vi "test.vi"() -> ()   [LabVIEW 2019]
uses:
  Settings.ctl
  <vilib>/DAQmx/write.llb/DAQmx Write (Analog DBL 1Chan 1Samp).vi
  <vilib>/DAQmx/create/channels.llb/DAQmx Create Channel (AO-Voltage-Basic).vi
  <vilib>/DAQmx/configure/timing.llb/DAQmx Timing (Sample Clock).vi
  <vilib>/DAQmx/miscellaneous.llb/DAQmx Fill In Error Info.vi
  <resource>/objmgr/daqmx.rc
panel:
  in  "rate":dbl=1000.0 format="%0.2f"
  in  "stop":bool
  in  "Sampling Rate":T1 format="%#_9f"
  in  "# Samples in":T1 format="%#_9f"
  in  "Strength (V)":dbl=5.0
  in  "Delay End (ms)":i32=52
  in  "Delay (ms)":dbl=20.0
  in  "Width of pulse (ms)":dbl=70.0
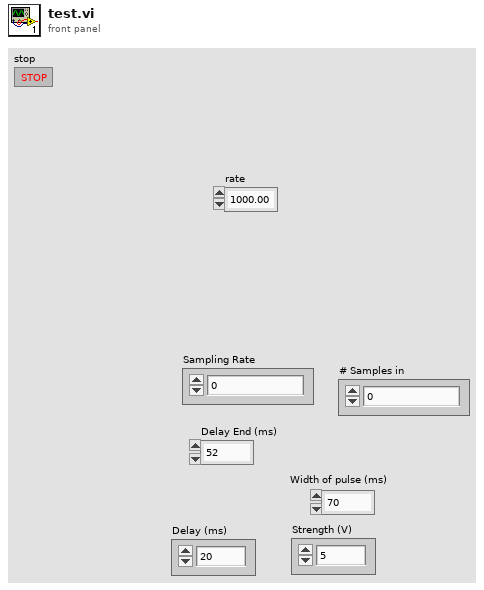
[diagram p1: front panel]
types:
  T1 = typedef "Settings.ctl" = dbl
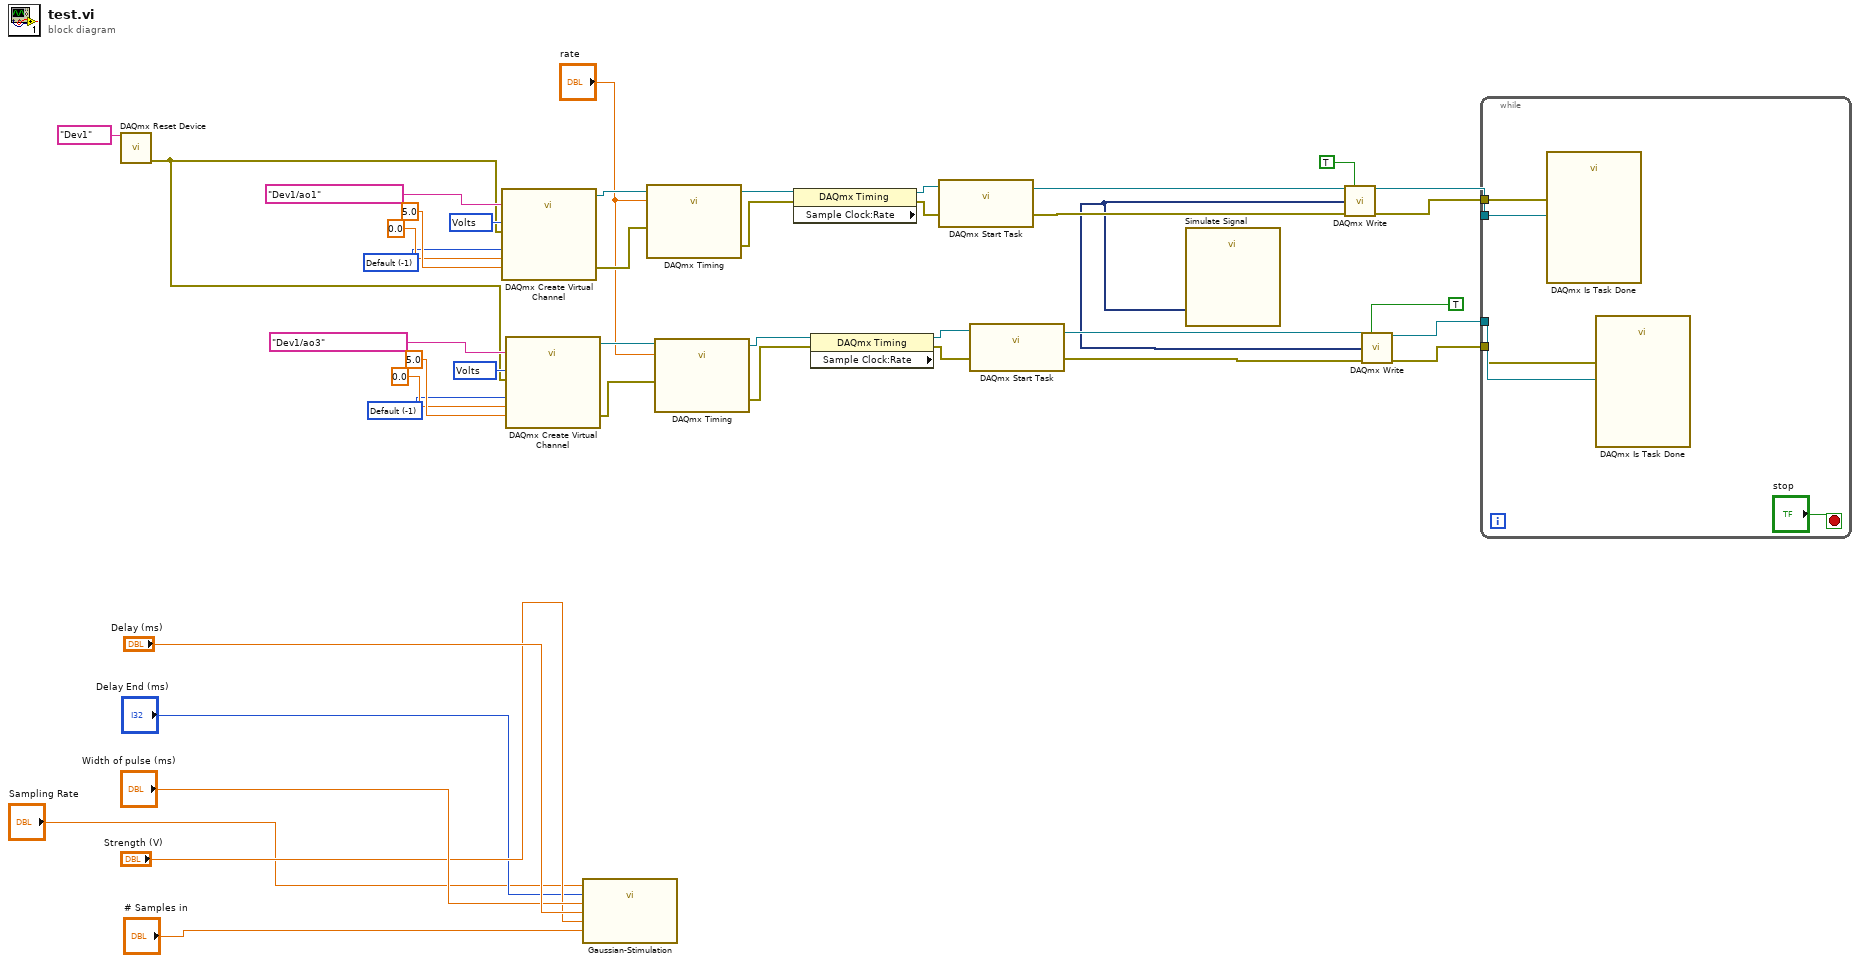
[diagram p0: block diagram]
diagram:
  w23 = 10348 items=["Volts"=10348, "From Custom Scale"=10065] ("units")
  w26 = -1 items=["Default"=-1, "RSE"=10083, "Differential"=10106, "Pseudodifferential"=12529] ("output terminal configuration")
  w36 = 10348 items=["Volts"=10348, "From Custom Scale"=10065] ("units")
  w39 = -1 items=["Default"=-1, "RSE"=10083, "Differential"=10106, "Pseudodifferential"=12529] ("output terminal configuration")
  n1 = call <vilib>:"DAQmx Reset Device.vi"("device in"=tag "Dev1") -> ("error out"=w22:errorcluster)  [unwired: 14 in]
  n2 = call-poly <vilib>:"DAQmx Create Virtual Channel.vi"("maximum value"=5.0, "minimum value"=0.0, "output terminal configuration"=w26, "physical channels"=tag "Dev1/ao1", "units"=w23, "error in"=w22) -> ("task out"=w15:refnum<k21>, "error out"=w14:errorcluster)  [unwired: 8 in]
  n3 = call-poly <vilib>:"DAQmx Create Virtual Channel.vi"("maximum value"=5.0, "minimum value"=0.0, "output terminal configuration"=w39, "physical channels"=tag "Dev1/ao3", "units"=w36, "error in"=w22) -> ("task out"=w9:refnum<k21>, "error out"=w8:errorcluster)  [unwired: 8 in]
  n4 = call "Gaussian-Stimulation.vi"("Strength (V)"="Strength (V)", "Delay (ms)"="Delay (ms)", "# Samples in"="# Samples in", "Width of pulse (ms)"="Width of pulse (ms)", "Delay End (ms)"="Delay End (ms)", "Sampling Rate"="Sampling Rate") -> ()  [unwired: 1 in, 5 out]
  n5 = call-poly <vilib>:"DAQmx Timing.vi"("task/channels in"=w15, "rate"="rate", "error in"=w14) -> ("task out"=w13:refnum<k21>, "error out"=w12:errorcluster)  [unwired: 4 in, 7 out]
  n6 = call-poly <vilib>:"DAQmx Timing.vi"("task/channels in"=w9, "rate"="rate", "error in"=w8) -> ("task out"=w7:refnum<k21>, "error out"=w6:errorcluster)  [unwired: 4 in, 7 out]
  n7 = property class="DAQmx Timing" props=["Sample Clock:Rate"](reference=w13, error in=w12) -> (reference out=w11:refnum<k21>, error out=w10:errorcluster)  [unwired: 1 out]
  n8 = property class="DAQmx Timing" props=["Sample Clock:Rate"](reference=w7, error in=w6) -> (reference out=w5:refnum<k21>, error out=w4:errorcluster)  [unwired: 1 out]
  n9 = call <vilib>:"DAQmx Start Task.vi"("task/channels in"=w11, "error in"=w10) -> ("task out"=w25:refnum<k21>, "error out"=w24:errorcluster)  [unwired: 12 in]
  n10 = call <vilib>:"DAQmx Start Task.vi"("task/channels in"=w5, "error in"=w4) -> ("task out"=w38:refnum<k21>, "error out"=w37:errorcluster)  [unwired: 12 in]
  n11 = call "Simulate Signal"() -> ("Sine"=w20:dynamicdata)  [unwired: 6 in, 9 out]
  n12 = call-poly <vilib>:"DAQmx Write.vi"("task/channels in"=w25, "auto start"=TRUE, "data"=w20, "error in"=w24) -> ("task out"=w17:refnum<k21>, "error out"=w16:errorcluster)  [unwired: 9 in, 1 out]
  n13 = call-poly <vilib>:"DAQmx Write.vi"("task/channels in"=w38, "auto start"=TRUE, "data"=w20, "error in"=w37) -> ("task out"=w3:refnum<k21>, "error out"=w2:errorcluster)  [unwired: 9 in, 1 out]
  n14 = while {
    tunnel: w17 -> [w47]
    tunnel: w16 -> [w46]
    tunnel: w3 -> [w45]
    tunnel: w2 -> [w44]
    stop <- "stop" stop-if-true
    n15 = call <vilib>:"DAQmx Is Task Done.vi"("task/channels in"=w47, "error in"=w46) -> ()  [unwired: 11 in, 3 out]
    n16 = call <vilib>:"DAQmx Is Task Done.vi"("task/channels in"=w45, "error in"=w44) -> ()  [unwired: 11 in, 3 out]
  }
